vi "CreateFolder.vi"(8 "error in (no error)":errorcluster, 10 "Path_Folder":path) -> (0 "error out":errorcluster, 2 "Path_Out":path)   [LabVIEW 2018]
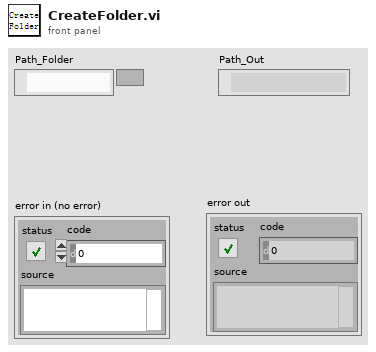
[diagram p1: front panel]
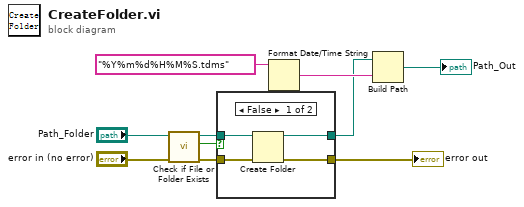
[diagram p0: block diagram]
diagram:
  n1 = call <vilib>:"Check if File or Folder Exists.vi"("error in (no error)"="error in (no error)", "path"="Path_Folder") -> ("error out"=w7:errorcluster, "file or folder exists?"=w6:bool, "dup path"=w5:path)  [unwired: 7 in]
  n2 = case shown="False" w6 {
    tunnel: w7 -> [w14 w16]
    tunnel: w5 -> [w13 w15]
    tunnel: [w12 w16] -> w4
    tunnel: [w11 w15] -> w1
    frame False {
      n3 = Create Folder(path (use dialog)=w13, error in=w14) -> (created path=w11:path, error out=w12:errorcluster)  [unwired: 1 in, 1 out]
    }
    frame True {
    }
  }
  "error out" <- w4
  n4 = Format Date/Time String(time format string (%c)="%Y%m%d%H%M%S.tdms") -> (date/time string=w9:string)  [unwired: 2 in]
  n5 = Build Path(base path=w1, name or relative path=w9) -> (appended path=→"Path_Out":path)
